vi "Configure Trigger Source [TRG].vi"(8 "error in (no error)":errorcluster, 9 "source (Immediate)":i32(ring) items=["Immediate", "External", "Software", "TTL0", "TTL1", "TTL2", "TTL3", "TTL4", "TTL5", "TTL6", "TTL7", "ECL0", "ECL1", "PXI Star", "RTSI 0", "RTSI 1", "RTSI 2", "RTSI 3", "RTSI 4", "RTSI 5", "RTSI 6"], 10 "channel name (\"CHANNEL1\")":string="CHANNEL1", 11 "IVI_DCPwr in":refnum<class "IVI_DCPwr.lvclass">) -> (0 "error out":errorcluster, 3 "IVI_DCPwr out":refnum<class "IVI_DCPwr.lvclass">)   [LabVIEW 2013, in "IVI_DCPwr.lvlib" / "IVI_DCPwr.lvclass"]
doc: "This VI configures the trigger source to which the power supply responds after you call IviDCPwr Initiate [TRG]. When the power supply receives a trigger signal on the source you specify, it changes its current and voltage outputs.\n\nYou configure the triggered current and voltage outputs with the\nIviDCPwr Configure Triggered Current Limit [TRG] and \nIviDCPwr Configure Triggered Voltage Level [TRG] VIs. \n\nNotes:\n\n(1) This VI is part of the IviDCPwrTrigger [TRG] extension group."
uses:
  IVI_DCPwr.lvclass
  IVI_DCPwr.lvclass/IVI_DCPwr.ctl
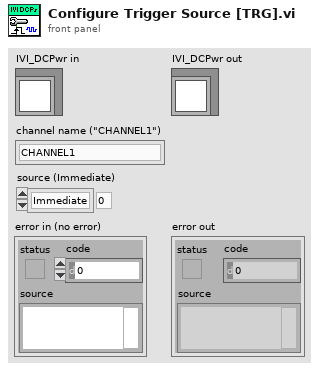
[diagram p1: front panel]
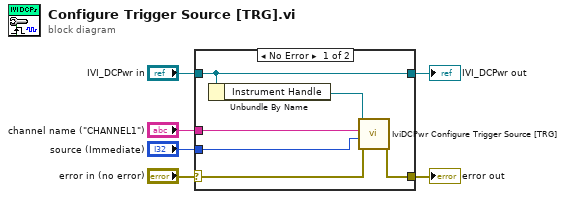
[diagram p0: block diagram]
diagram:
  n1 = case shown="No Error" "error in (no error)" {
    selector: "error in (no error)" -> [w10 w14]
    tunnel: [w9 w14] -> w5
    tunnel: [w12 w13] -> w3
    tunnel: "IVI_DCPwr in" -> [w12 w13]
    tunnel: "channel name (\"CHANNEL1\")" -> [w8 _]
    tunnel: "source (Immediate)" -> [w7 _]
    frame No Error {
      n2 = Unbundle By Name(w12) -> ("Instrument Handle"=w11:refnum<k15>)
      n3 = call <vilib>:"IviDCPwr Configure Trigger Source [TRG].vi"("error in (no error)"=w10, "source (Immediate)"=w7, "channel name (\"CHANNEL1\")"=w8, "instrument handle"=w11) -> ("error out"=w9:errorcluster)  [unwired: 6 in, 1 out]
    }
    frame Error {
    }
  }
  "error out" <- w5
  "IVI_DCPwr out" <- w3
